vi "AutoTurn.vi"(11 "Target Robot Angle":dbl) -> (1 "Done":bool)   [LabVIEW 2017]
uses:
  Robot Global Data.vi
  <vilib>/addons/control/pid/pid.llb/PID (DBL).vi
  <vilib>/addons/control/pid/NI_PID_pid.lvlib
panel:
  in  "Output On":bool=TRUE
  out "output":dbl format="%.2f"
  out "output array":bool[](array[boolean])
  in  "Allowable Angle Error":dbl=1.0
  out "output - Angle":dbl(graph)
  in  "PID gains - Angle":T1={"proportional gain (Kc)"=0.020000000000000007, "integral time (Ti, min)"=0.0, "derivative time (Td, min)"=0.005} {"derivative time (Td, min)" step=0.001 format="%.5f"; "integral time (Ti, min)" step=0.001 format="%.5f"; "proportional gain (Kc)" step=0.001 format="%.5f"}
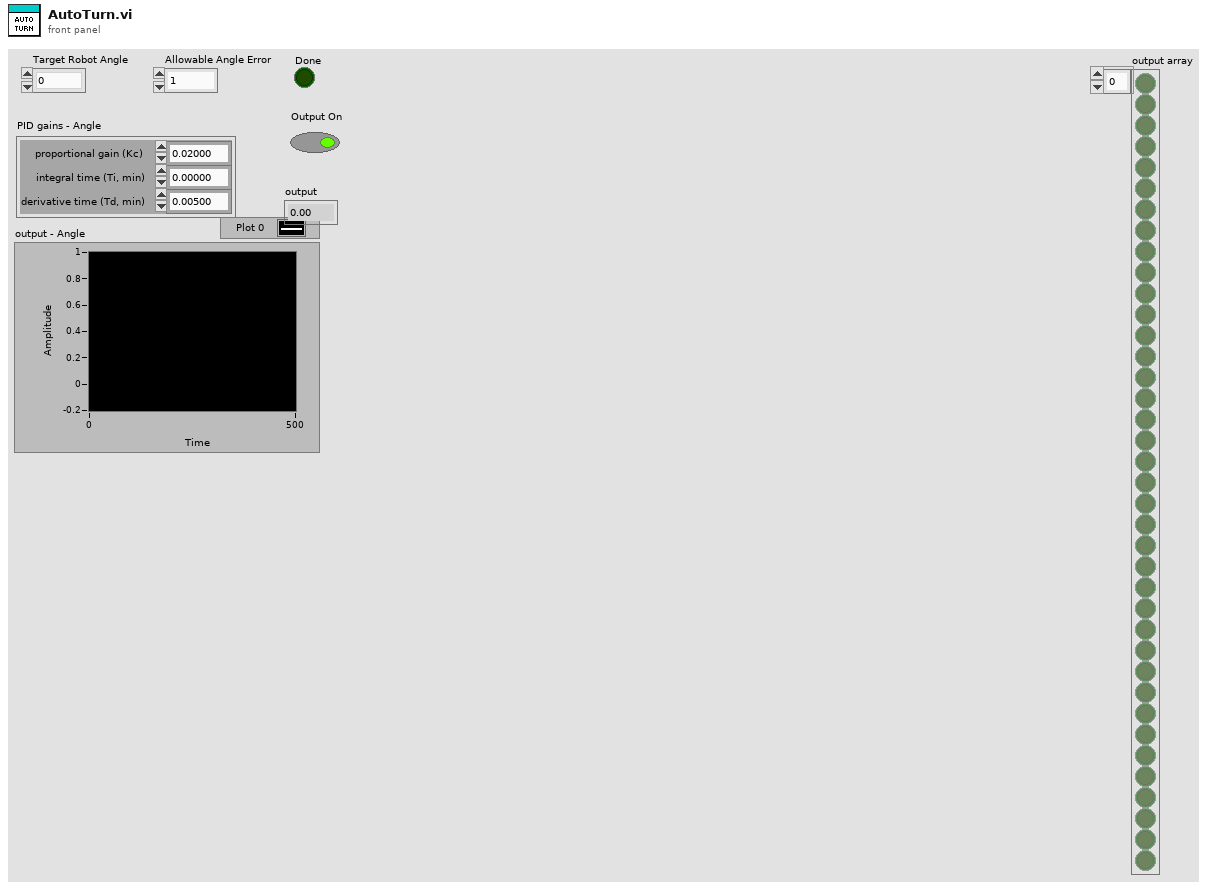
[diagram p1: front panel]
types:
  T1 = cluster{"proportional gain (Kc)":dbl, "integral time (Ti, min)":dbl, "derivative time (Td, min)":dbl}
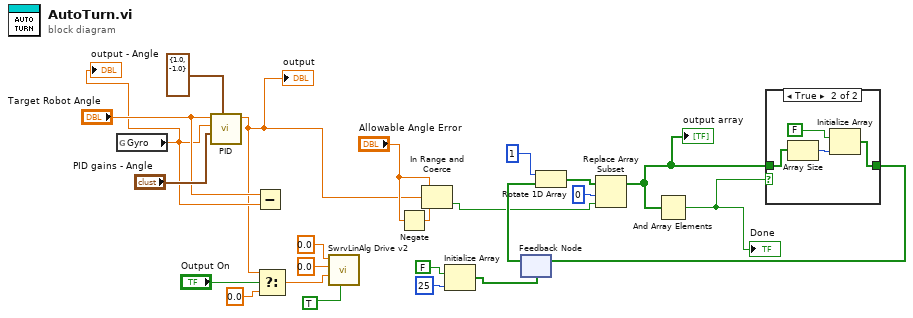
[diagram p0: block diagram]
diagram:
  n1 = global read "Robot Global Data.vi" "Gyro"() -> (w2:dbl)
  "output - Angle" <- w2
  n2 = call-poly <vilib>:"PID.vi"("output range"=cluster{"output high":dbl, "output low":dbl} {"output high"=1.0, "output low"=-1.0}, "PID gains"="PID gains - Angle", "process variable"=w2, "setpoint"="Target Robot Angle") -> ("output"=w1:dbl)  [unwired: 6 in, 1 out]
  "output" <- w1
  n3 = Subtract(x="Target Robot Angle", y=w2) -> ()  [unwired: 1 out]
  n4 = Select(t=w1, s="Output On", f=0.0) -> (s? t:f=w4:dbl)
  n5 = call "SwrvLinAlg Drive v2.vi"("Auto Controls"=TRUE, "Z"=w4, "Y"=0.0, "X"=0.0) -> ()  [unwired: 8 in]
  n6 = Negate(x="Allowable Angle Error") -> (-x=w22:dbl)
  n7 = In Range and Coerce(upper limit="Allowable Angle Error", x=w1, lower limit=w22) -> (In Range?=w12:bool)  [unwired: 1 out]
  n8 = Initialize Array(FALSE, 25 ("dimension size")) -> (w9:bool[])
  n9 = feedback #1(w9) -> (w14:bool[])
  n10 = Rotate 1D Array(1:w14, 2:1 ("n")) -> (0:w16:bool[])
  n11 = Replace Array Subset(array=w16, new element=w12, index=0) -> (w11:bool[])
  "output array" <- w11
  n12 = And Array Elements(Boolean array=w11) -> (logical AND=w10:bool)
  "Done" <- w10
  n13 = case shown="True" w10 {
    tunnel: w11 -> [w25 w27]
    tunnel: [w25 w26] -> w13
    frame False {
    }
    frame True {
      n14 = Array Size(array=w27) -> (size(s)=w28:i32)
      n15 = Initialize Array(FALSE, w28) -> (w26:bool[])
    }
  }
  n16 = feedback-in #1(w13) -> ()
